vi "SAOMM-SetTelescopeProperties.vi"(0 "PRAMMS-COMM IN":refnum<visa-resource-name>="Hp\u0000\u0002", 1 "PramsActif":refnum<vi>, 2 "PrAMS-ACK":refnum<vi>, 5 "HA":dbl, 7 "DEC":dbl, 11 "Error IN":errorcluster, 12 "Signature":u32=1886544237, 13 "MsgTypeEnum":cluster{"Type":string[], "Enum":u32[]}={"Type"=["emtError", "emtAreYouThere", "emtAcknowledgment", "emtGetClientType", "emtClientType", "emtGetImageExposureTime", "emtSetImageExposureTime", "emtImageExposureTime", "emtGetOptimalExposureTime", "emtSetOptimalExposureTime", "emtOptimalExposureTime", "emtGetImageEMGain", "emtSetImageEMGain", "emtImageEMGain", "emtGetFPGACtrl", "emtSetFPGACtrl", "emtFPGACtrl", "emtGetImageWidth", "emtSetImageWidth", "emtImageWidth", "emtGetImageHeight", "emtSetImageHeight", "emtImageHeight", "emtGetImageBinning", "emtSetImageBinning", "emtImageBinning", "emtGetImageDisplayFrameRate", "emtSetImageDisplayFrameRate", "emtImageDisplayFrameRate", "emtGetROIWidth", "emtSetROIWidth", "emtROIWidth", "emtGetROIHeight", "emtSetROIHeight", "emtROIHeight", "emtGetROIXOffset", "emtSetROIXOffset", "emtROIXOffset", "emtGetROIYOffset", "emtSetROIYOffset", "emtROIYOffset", "emtStartAcquisition", "mtStopAcquisition", "emtAcquisitionStarted", "emtAcquisitionStopped", "emtGetFalconImage", "emtFalconImage"], "Enum"=[1, 2, 3, 4, 5, 1001, 1101, 1201, 1002, 1102, 1202, 1003, 1103, 1203, 1004, 1104, 1204, 1005, 1105, 1205, 1006, 1106, 1206, 1007, 1107, 1207, 1008, 1108, 1208, 1009, 1109, 1209, 1010, 1110, 1210, 1011, 1111, 1211, 1012, 1112, 1212, 1130, 1131, 1150, 1151, 1070, 1270]}) -> (4 "PRAMMS-COMM OUT":refnum<visa-resource-name>, 15 "Error OUT":errorcluster)   [LabVIEW 2019]
uses:
  Polymorphics/Num2littleEndian(DBL).vi
panel:
  out "AZ":dbl
  out "ALT":dbl
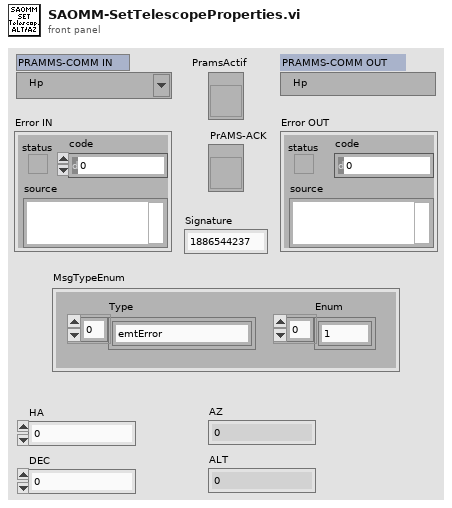
[diagram p1: front panel]
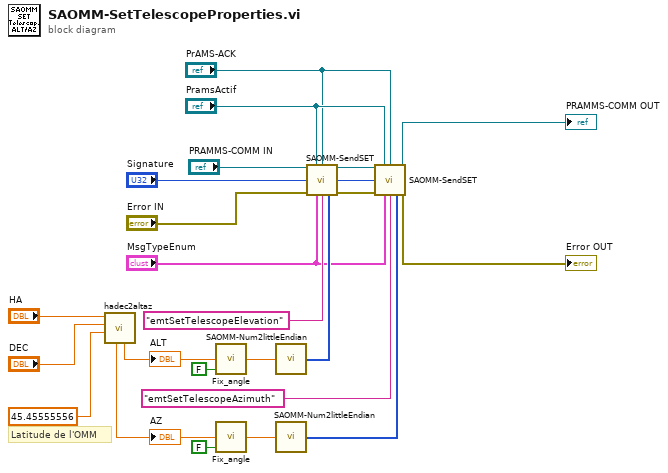
[diagram p0: block diagram]
diagram:
  # "Latitude de l'OMM"
  n1 = call "hadec2altaz.vi"("LAT"=45.45555556, "DEC"="DEC", "HA"="HA") -> ("Alt (theta)"=w14:dbl, "Az (phi)"=w8:dbl)  [unwired: 4 in, 3 out]
  "ALT" <- w14
  "AZ" <- w8
  n2 = call "Fix_angle.vi"("±180 -> 0-360?"=FALSE, "Angle IN"=w14) -> ("Angle OUT"=w11:dbl)  [unwired: 3 in]
  n3 = call "Fix_angle.vi"("±180 -> 0-360?"=FALSE, "Angle IN"=w8) -> ("Angle OUT"=w7:dbl)  [unwired: 3 in]
  n4 = call-poly "SAOMM-Num2littleEndian.vi"("Number"=w11) -> ("LiitleEndianedData"=w13:u8[])  [unwired: 14 in]
  n5 = call-poly "SAOMM-Num2littleEndian.vi"("Number"=w7) -> ("LiitleEndianedData"=w12:u8[])  [unwired: 14 in]
  n6 = call "SAOMM-SendSET.vi"("PRAMMS-COMM IN"="PRAMMS-COMM IN", "Active Refnum"="PramsActif", "PrAMS-ACK"="PrAMS-ACK", "Signature"="Signature", "Error IN"="Error IN", "MessageType"="MsgTypeEnum", "Active SET"="emtSetTelescopeElevation", "Value (little endianed byte array)"=w13) -> ("PRAMMS-COMM OUT"=w21:refnum<visa-resource-name>, "Error OUT"=w20:errorcluster)  [unwired: 4 in, 2 out]
  n7 = call "SAOMM-SendSET.vi"("PRAMMS-COMM IN"=w21, "Active Refnum"="PramsActif", "PrAMS-ACK"="PrAMS-ACK", "Signature"="Signature", "Error IN"=w20, "MessageType"="MsgTypeEnum", "Active SET"="emtSetTelescopeAzimuth", "Value (little endianed byte array)"=w12) -> ("PRAMMS-COMM OUT"=→"PRAMMS-COMM OUT":refnum<visa-resource-name>, "Error OUT"=→"Error OUT":errorcluster)  [unwired: 4 in, 2 out]
